vi "PH_AxisGUI_NF2.ProcCases.vi"(0 "i ref in":refnum<vi>, 1 "selector":string, 2 "data":i8[](array[numeric]), 3 "call cluster":T1={"Object"="", "Selector"="", "CallType"=enum."synchronous", "Async Object"="", "Async Selector"="", "Data Descriptor"="", "Data"=[], "Error #"=0, "Expire"=0}, 5 "error in":errorcluster) -> (14 "i ref out":refnum<vi>, 17 "answer cluster":T1={"Object"="", "Selector"="", "CallType"=enum."synchronous", "Async Object"="", "Async Selector"="", "Data Descriptor"="", "Data"=[], "Error #"=0, "Expire"=0}, 19 "error out":errorcluster)   [LabVIEW 2014, in "PH_AxisGUI_NF2.lvlib"]
doc: "This method is called by a process from within the default case in the event loop. The methods of a class that are linked to events will be called from THIS method. Add your code here."
uses:
  PH_AxisGUI_NF2.lvlib
  CS_Core/CSSystem/CoreDefs/CoreDefs.call_type.ctl
  CS_Core/BaseProcess/BaseProcess.descriptor string definition.ctl
  CS_Core/CSSystem/CoreDefs/CoreDefs.rawDataType.ctl
  CS_Core/CSSystem/CoreLib/CoreLib.string 2 byte array.vi
  CS_Core/CSSystem/CoreLib/CoreLib.byte array 2 int.vi
  CS_Core/BaseProcess/BaseProcess.lvlib
  CS_Core/CSSystem/CoreLib/CoreLib.lvlib
  PH_Basics/PH_StatusHandler/PH_StatusHandler.lvlib
  CS_Core/CAEObj/CAEObj.lvlib
  PH_Basics/PH_Common/PH_Common.lvlib
  PH_Basics/PH_Class/PH_Class.lvlib
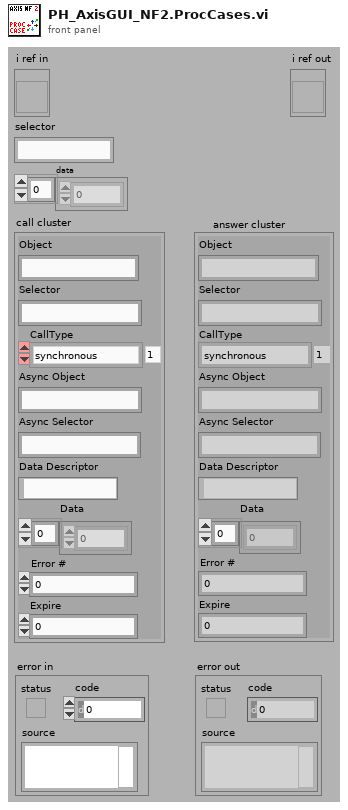
[diagram p1: front panel]
types:
  T1 = typedef "CoreDefs.call_type.ctl" = cluster{"Object":string, "Selector":string, "CallType":enum16{"simple", "synchronous", "asynchronous"}, "Async Object":string, "Async Selector":string, "Data Descriptor":T2, "Data":T3, "Error #":i32, "Expire":u32}
  T2 = typedef "BaseProcess.lvlib/BaseProcess.descriptor string definition.ctl" = string
  T3 = typedef "CoreDefs.rawDataType.ctl" = i8[]
  T4 = typedef "PH_StatusHandler.lvlib/PH_StatusHandler.Status.ctl" = i16
  T5 = typedef "PH_AxisGUI_NF2.lvlib/PH_AxisGUI_NF2.i attribute.ctl" = cluster{"GUI Refs":cluster{"Delete":refnum<vi>, "Instance Status":refnum<vi>, "Width Axis 1":refnum<vi>, "Width Axis 2":refnum<vi>}, "Instance":string, "System":string, "Width Axis 1":i32, "Width Axis 2":i32, "Sign Change Axis 1":bool, "Sign Change Axis 2":bool, "Motor Axis 1":i32, "Motor Axis 2":i32}
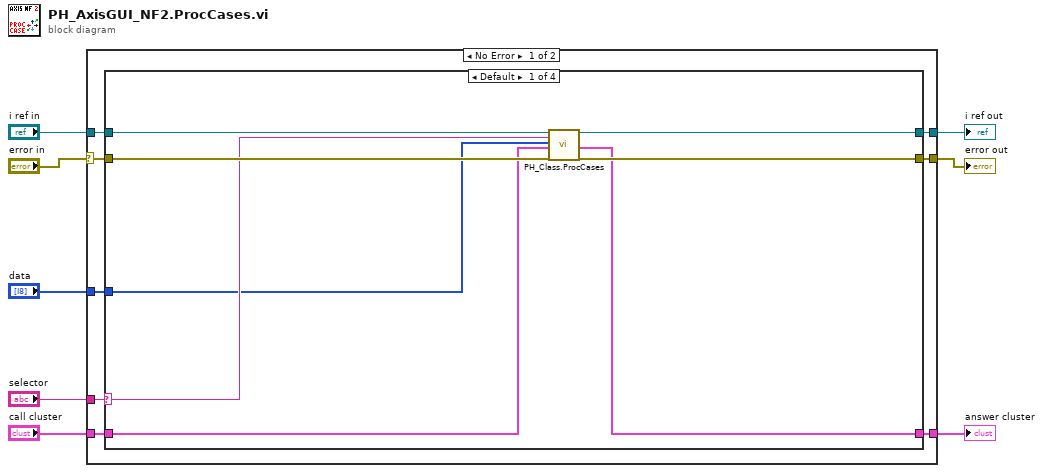
[diagram p0: block diagram]
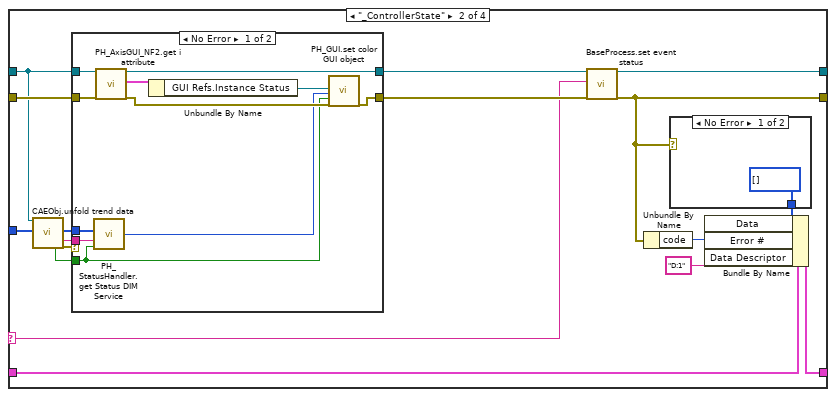
[diagram p2: hidden frame]
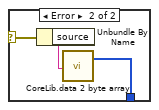
[diagram p3: hidden frame]
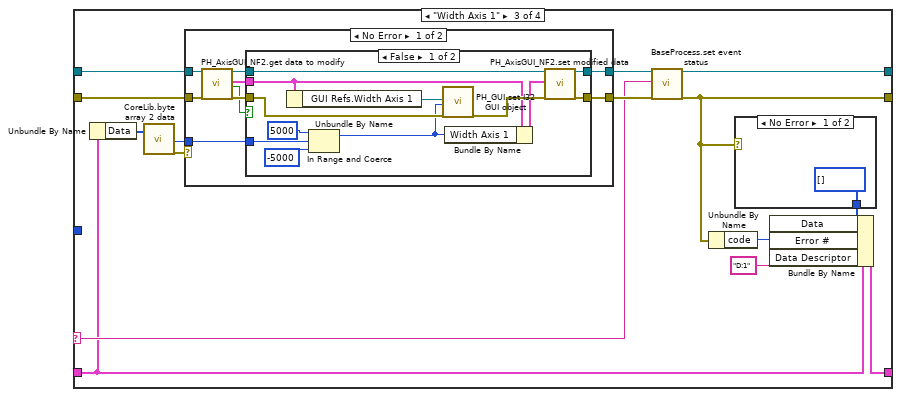
[diagram p5: hidden frame]
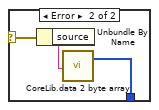
[diagram p6: hidden frame]
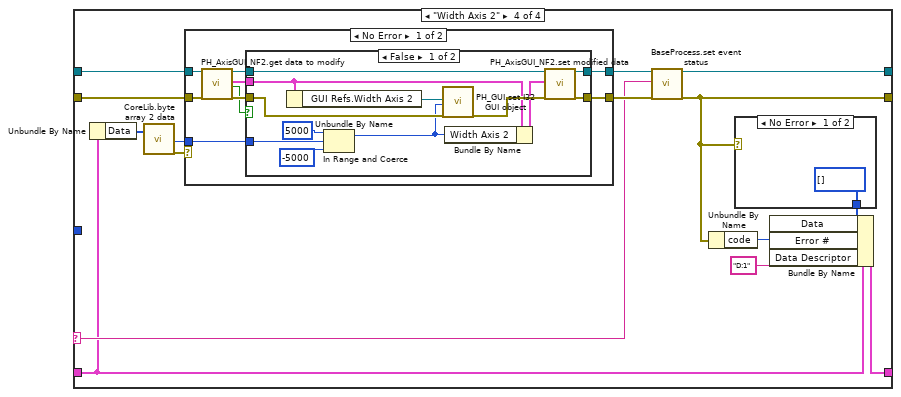
[diagram p9: hidden frame]
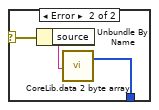
[diagram p10: hidden frame]
diagram:
  n1 = case shown="No Error" "error in" {
    selector: "error in" -> [w10 w148]
    tunnel: "selector" -> [w16 _]
    tunnel: [w15 w147] -> w7
    tunnel: "call cluster" -> [w14 w147]
    tunnel: "i ref in" -> [w13 w149]
    tunnel: [w12 w149] -> w4
    tunnel: [w9 w148] -> w3
    tunnel: "data" -> [w11 _]
    frame No Error {
      n2 = case shown="Default" w16 {
        selector: w16 -> [w19 w38 w70 w114]
        tunnel: w13 -> [w18 w31 w64 w108]
        tunnel: [w24 w37 w69 w113] -> w12
        tunnel: w14 -> [w20 w26 w61 w105]
        tunnel: [w21 w25 w63 w107] -> w15
        tunnel: w10 -> [w23 w41 w73 w117]
        tunnel: w11 -> [w17 w32 _ _]
        tunnel: [w22 w33 w65 w109] -> w9
        frame Default {
          n3 = call "PH_Class.ProcCases.vi"("i ref in"=w18, "selector"=w19, "Data"=w17, "call cluster"=w20, "error in (no error)"=w23) -> ("i ref out"=w24:refnum<vi>, "answer cluster"=w21:T1, "error out"=w22:errorcluster)  [unwired: 12 in]
        }
        frame "_ControllerState" {
          n4 = call "CAEObj.unfold trend data.vi"("i ref in"=w31, "raw trend data"=w32) -> ("no link"=w27:bool, "data"=w29:i8[], "typeDescriptor"=w28:string, "error out"=w30:errorcluster)  [unwired: 9 in, 5 out]
          n5 = case shown="No Error" w30 {
            tunnel: [w53 w58] -> w40
            tunnel: w31 -> [w54 w58]
            tunnel: w41 -> [w52 w57]
            tunnel: [w48 w57] -> w39
            tunnel: w29 -> [w56 _]
            tunnel: w28 -> [w55 _]
            tunnel: w27 -> [w47 _]
            frame No Error {
              n6 = call "PH_StatusHandler.get Status DIM Service.vi"("no link"=w47, "typeDescriptor"=w55, "data"=w56) -> ("Status"=w46:T4)  [unwired: 1 in]
              n7 = call "PH_AxisGUI_NF2.get i attribute.vi"("i ref in"=w54, "error in (no error)"=w52) -> ("i ref out"=w53:refnum<vi>, "i attribute"=w51:T5, "error out"=w49:errorcluster)  [unwired: 15 in]
              n8 = Unbundle By Name(w51) -> ("GUI Refs.Instance Status"=w50:refnum<vi>)
              n9 = call "PH_GUI.set color GUI object.vi"("GUI object Ref"=w50, "State"=w46, "Blinking? (false)"=w47, "error in (no error)"=w49) -> ("error out"=w48:errorcluster)  [unwired: 15 in]
            }
            frame Error {
            }
          }
          n10 = call "BaseProcess.set event status.vi"("i ref in"=w40, "EventStatus"=w38, "error in (no error)"=w39) -> ("i ref out"=w37:refnum<vi>, "error out"=w33:errorcluster)  [unwired: 14 in, 1 out]
          n11 = Unbundle By Name(w33) -> ("code"=w36:i32)
          n12 = case shown="No Error" w33 {
            selector: w33 -> [_ w45]
            tunnel: [T3 [] ("byteArray out") w43] -> w34
            frame No Error {
            }
            frame Error {
              n13 = Unbundle By Name(w45) -> ("source"=w44:string)
              n14 = call-poly "CoreLib.data 2 byte array.vi"("string"=w44) -> ("byteArray out"=w43:T3)  [unwired: 18 in]
            }
          }
          n15 = Bundle By Name(cluster=w26, "Data"=w34, "Error #"=w36, "Data Descriptor"="D:1") -> (w25:T1)
        }
        frame "Width Axis 1" {
          n16 = Unbundle By Name(w61) -> ("Data"=w62:T3)
          n17 = call-poly "CoreLib.byte array 2 data.vi"("byteArray"=w62) -> ("i32"=w59:i32, "error out"=w60:errorcluster)  [unwired: 16 in, 1 out]
          n18 = case shown="No Error" w60 {
            tunnel: [w82 w102] -> w72
            tunnel: w64 -> [w86 w102]
            tunnel: w73 -> [w85 w101]
            tunnel: [w81 w101] -> w71
            tunnel: w59 -> [w79 _]
            frame No Error {
              n19 = call "PH_AxisGUI_NF2.get data to modify.vi"("i ref in"=w86, "error in (no error)"=w85) -> ("i ref out"=w83:refnum<vi>, "i attribute"=w80:T5, "timed out"=w78:bool, "error out"=w84:errorcluster)  [unwired: 14 in]
              n20 = case shown="False" w78 {
                tunnel: w84 -> [w97 w99]
                tunnel: w83 -> [w96 w100]
                tunnel: [w95 w100] -> w82
                tunnel: [w93 w99] -> w81
                tunnel: w80 -> [w92 _]
                tunnel: w79 -> [w90 _]
                frame False {
                  n21 = Unbundle By Name(w92) -> ("GUI Refs.Width Axis 1"=w98:refnum<vi>)
                  n22 = In Range and Coerce(upper limit=5000, x=w90, lower limit=-5000) -> (coerced(x)=w89:i32)  [unwired: 1 out]
                  n23 = call "PH_GUI.set I32 GUI object.vi"("I32 GUI Ref"=w98, "value"=w89, "error in (no error)"=w97) -> ("error out"=w94:errorcluster)  [unwired: 16 in]
                  n24 = Bundle By Name(cluster=w92, "Width Axis 1"=w89) -> (w91:T5)
                  n25 = call "PH_AxisGUI_NF2.set modified data.vi"("i ref in"=w96, "i attribute"=w91, "error in (no error)"=w94) -> ("i ref out"=w95:refnum<vi>, "error out"=w93:errorcluster)  [unwired: 15 in]
                }
                frame True {
                }
              }
            }
            frame Error {
            }
          }
          n26 = call "BaseProcess.set event status.vi"("i ref in"=w72, "EventStatus"=w70, "error in (no error)"=w71) -> ("i ref out"=w69:refnum<vi>, "error out"=w65:errorcluster)  [unwired: 14 in, 1 out]
          n27 = Unbundle By Name(w65) -> ("code"=w68:i32)
          n28 = case shown="No Error" w65 {
            selector: w65 -> [_ w77]
            tunnel: [T3 [] ("byteArray out") w75] -> w66
            frame No Error {
            }
            frame Error {
              n29 = Unbundle By Name(w77) -> ("source"=w76:string)
              n30 = call-poly "CoreLib.data 2 byte array.vi"("string"=w76) -> ("byteArray out"=w75:T3)  [unwired: 18 in]
            }
          }
          n31 = Bundle By Name(cluster=w61, "Data"=w66, "Error #"=w68, "Data Descriptor"="D:1") -> (w63:T1)
        }
        frame "Width Axis 2" {
          n32 = Unbundle By Name(w105) -> ("Data"=w106:T3)
          n33 = call-poly "CoreLib.byte array 2 data.vi"("byteArray"=w106) -> ("i32"=w103:i32, "error out"=w104:errorcluster)  [unwired: 16 in, 1 out]
          n34 = case shown="No Error" w104 {
            tunnel: [w126 w146] -> w116
            tunnel: w108 -> [w130 w146]
            tunnel: w117 -> [w129 w145]
            tunnel: [w125 w145] -> w115
            tunnel: w103 -> [w123 _]
            frame No Error {
              n35 = call "PH_AxisGUI_NF2.get data to modify.vi"("i ref in"=w130, "error in (no error)"=w129) -> ("i ref out"=w127:refnum<vi>, "i attribute"=w124:T5, "timed out"=w122:bool, "error out"=w128:errorcluster)  [unwired: 14 in]
              n36 = case shown="False" w122 {
                tunnel: w128 -> [w141 w143]
                tunnel: w127 -> [w140 w144]
                tunnel: [w139 w144] -> w126
                tunnel: [w137 w143] -> w125
                tunnel: w124 -> [w136 _]
                tunnel: w123 -> [w132 _]
                frame False {
                  n37 = Unbundle By Name(w136) -> ("GUI Refs.Width Axis 2"=w142:refnum<vi>)
                  n38 = In Range and Coerce(upper limit=5000, x=w132, lower limit=-5000) -> (coerced(x)=w131:i32)  [unwired: 1 out]
                  n39 = call "PH_GUI.set I32 GUI object.vi"("I32 GUI Ref"=w142, "value"=w131, "error in (no error)"=w141) -> ("error out"=w138:errorcluster)  [unwired: 16 in]
                  n40 = Bundle By Name(cluster=w136, "Width Axis 2"=w131) -> (w135:T5)
                  n41 = call "PH_AxisGUI_NF2.set modified data.vi"("i ref in"=w140, "i attribute"=w135, "error in (no error)"=w138) -> ("i ref out"=w139:refnum<vi>, "error out"=w137:errorcluster)  [unwired: 15 in]
                }
                frame True {
                }
              }
            }
            frame Error {
            }
          }
          n42 = call "BaseProcess.set event status.vi"("i ref in"=w116, "EventStatus"=w114, "error in (no error)"=w115) -> ("i ref out"=w113:refnum<vi>, "error out"=w109:errorcluster)  [unwired: 14 in, 1 out]
          n43 = Unbundle By Name(w109) -> ("code"=w112:i32)
          n44 = case shown="No Error" w109 {
            selector: w109 -> [_ w121]
            tunnel: [T3 [] ("byteArray out") w119] -> w110
            frame No Error {
            }
            frame Error {
              n45 = Unbundle By Name(w121) -> ("source"=w120:string)
              n46 = call-poly "CoreLib.data 2 byte array.vi"("string"=w120) -> ("byteArray out"=w119:T3)  [unwired: 18 in]
            }
          }
          n47 = Bundle By Name(cluster=w105, "Data"=w110, "Error #"=w112, "Data Descriptor"="D:1") -> (w107:T1)
        }
      }
    }
    frame Error {
    }
  }
  "answer cluster" <- w7
  "i ref out" <- w4
  "error out" <- w3
